vi "Result.StatusStr to Integer.vi"(11 "StatusStr":string) -> (3 "Status":T1 items=["LOG", "PASS", "FAIL", "ERROR"])   [LabVIEW 2018]
uses:
  Result.Measurement and Attribute Item Status.ctl
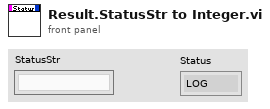
[diagram p1: front panel]
types:
  T1 = typedef "Result.Measurement and Attribute Item Status.ctl" = i32
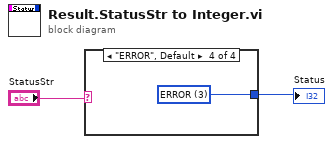
[diagram p0: block diagram]
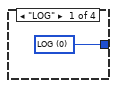
[diagram p2: hidden frame]
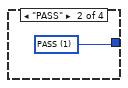
[diagram p3: hidden frame]
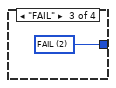
[diagram p4: hidden frame]
diagram:
  n1 = case shown="\"ERROR\", Default" "StatusStr" {
    tunnel: [w3 w4 w5 w6] -> w1
    frame "LOG" {
      w3 = T1 0 items=["LOG", "PASS", "FAIL", "ERROR"] ("Status")
    }
    frame "PASS" {
      w4 = T1 1 items=["LOG", "PASS", "FAIL", "ERROR"] ("Status")
    }
    frame "FAIL" {
      w5 = T1 2 items=["LOG", "PASS", "FAIL", "ERROR"] ("Status")
    }
    frame "ERROR", Default {
      w6 = T1 3 items=["LOG", "PASS", "FAIL", "ERROR"] ("Status")
    }
  }
  "Status" <- w1
